vi "Cleanup.vi"(8 "error in (no error)":errorcluster, 11 "BetterSearch in":refnum<class "BetterSearch.lvclass">) -> (0 "error out":errorcluster)   [LabVIEW 2020, in "Better Search.lvlib" / "BetterSearch.lvclass"]
uses:
  BetterSearch.lvclass
  BetterSearch.lvclass/BetterSearch.ctl
  Search/Search.lvclass
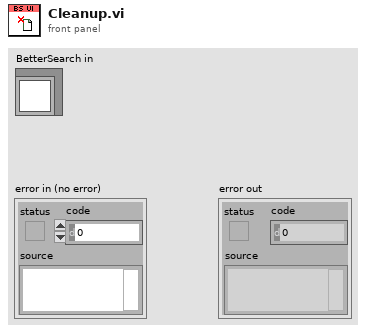
[diagram p1: front panel]
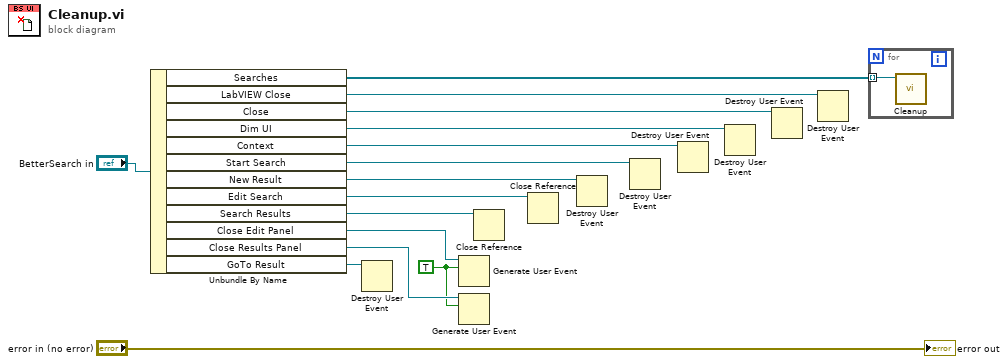
[diagram p0: block diagram]
diagram:
  w6 = TRUE ("event data")
  n1 = Unbundle By Name("BetterSearch in") -> ("Searches"=w5:refnum<class "Search.lvclass">[], "LabVIEW Close"=w2:refnum<user-event>, "Close"=w3:refnum<user-event>, "Dim UI"=w4:refnum<user-event>, "Context"=w11:refnum<user-event>, "Start Search"=w12:refnum<user-event>, "New Result"=w13:refnum<user-event>, "Edit Search"=w9:refnum<vi>, "Search Results"=w10:refnum<vi>, "Close Edit Panel"=w8:refnum<user-event>, "Close Results Panel"=w7:refnum<user-event>, "GoTo Result"=w1:refnum<user-event>)
  n2 = Destroy User Event(user event=w1) -> ()  [unwired: 1 in, 1 out]
  n3 = Generate User Event(user event=w8, event data cluster=w6) -> ()  [unwired: 2 in, 2 out]
  n4 = Generate User Event(user event=w7, event data cluster=w6) -> ()  [unwired: 2 in, 2 out]
  n5 = Close Reference(reference=w10) -> ()  [unwired: 1 in, 1 out]
  n6 = Close Reference(reference=w9) -> ()  [unwired: 1 in, 1 out]
  n7 = Destroy User Event(user event=w13) -> ()  [unwired: 1 in, 1 out]
  n8 = Destroy User Event(user event=w12) -> ()  [unwired: 1 in, 1 out]
  n9 = Destroy User Event(user event=w11) -> ()  [unwired: 1 in, 1 out]
  n10 = Destroy User Event(user event=w4) -> ()  [unwired: 1 in, 1 out]
  n11 = Destroy User Event(user event=w3) -> ()  [unwired: 1 in, 1 out]
  n12 = Destroy User Event(user event=w2) -> ()  [unwired: 1 in, 1 out]
  n13 = for {
    tunnel: w5 -> [w16] mode=indexing
    n14 = call "Cleanup.vi"("Search in"=w16) -> ()  [unwired: 10 in, 1 out]
  }
  "error out" <- "error in (no error)"
